vi "Reset Server Information.vi"(8 "error in (no error)":errorcluster, 11 "System Information Controls In":refnum<vi>[](array[refnum])) -> (0 "error out":errorcluster, 3 "System Information Controls Out":refnum<vi>[](array[refnum]))   [LabVIEW 2024]
doc: "Resets the server information controls."
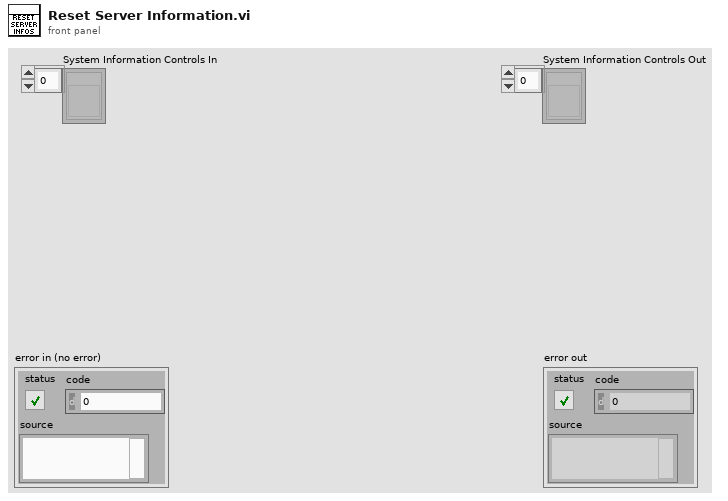
[diagram p1: front panel]
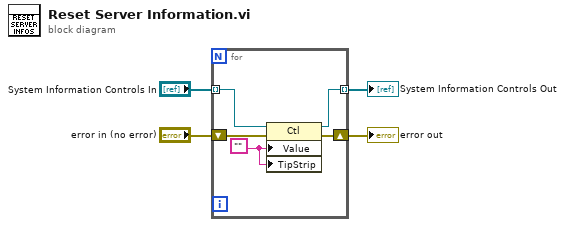
[diagram p0: block diagram]
diagram:
  n1 = for {
    tunnel: "System Information Controls In" -> [w9] mode=indexing
    shift-right: [w6] -> w1
    shift-left: "error in (no error)" -> [w8]
    tunnel: [w7] -> w3 mode=indexing
    w5 = "" ("Value")
    n2 = property class="Ctl"(reference=w9, error in=w8, "Value"=w5, "TipStrip"=w5) -> (reference out=w7:refnum<vi>, error out=w6:errorcluster)
  }
  "error out" <- w1
  "System Information Controls Out" <- w3
